vi "soundwave_generator_v06_complete_main.vi"() -> ()   [LabVIEW 2019]
uses:
  controls/Data.ctl
  <vilib>/sound2/lvsound2.llb/Sound Output Task ID.ctl
  controls/State.ctl
  <vilib>/sound2/lvsound2.llb/Sound Data Format.ctl
  <vilib>/sound2/lvsound2.llb/Sampling Mode.ctl
  <vilib>/Platform/TimedLoop/XDataNode/timing_clust.ctl
  <vilib>/Platform/TimedLoop/XDataNode/nitl_modes.ctl
  <vilib>/Platform/TimedLoop/XDataNode/wakeup.ctl
  add63f69-d936-4ba7-9212-3bb4b78ce241.vi
  global.vi
  <vilib>/sound2/lvsound2.llb/Sound File Read Open.vi
  <vilib>/sound2/lvsound2.llb/Sound File Read (DBL).vi
  <vilib>/Waveform/WDTOps.llb/WDT Waveform Duration DBL.vi
  <vilib>/sound2/lvsound2.llb/Sound Output Set Volume (Single).vi
  <vilib>/sound2/lvsound2.llb/Sound Output Write (DBL Single).vi
  <vilib>/platform/TimedLoop/XDataNode/XDataNode.xnode
  <vilib>/Platform/TimedLoop/XDataNode/XDNodeRunTimeDep.lvlib
panel:
  in  "Waiting time 2 [ms]":i32=1000
  in  "Waiting time 1 [ms]":i32=2000
  in  "# Repetitions":i32=3
  out "User Choice":string
  out "Real sound Duration [s] (Not Rounded)":dbl
  in  "Volume":dbl(slide)=50.0 min=0.0 max=100.0 step=1.0 scale=0.0..100.0
  out "Sound Duration [s]":dbl
  in  "Sound Samples Directory":path=path "D:/Scuola Superiore Sant'Anna/Neuro-Robotic Touch Laboratory - PhD Marian Statache - PhD Marian Statache/03 - HW & SW/Sound Psychophysical Protocol v3/sound_samples/2sec_352-00_396-00_412-50_440-00_469-33_495-00_528-00" caption="start path"
  out "Section 5":bool
  out "Section 4":bool
  out "Section 3":bool
  out "Section 1":bool
  in  "Saving Directory":path=path "D:/Scuola Superiore Sant'Anna/Neuro-Robotic Touch Laboratory - PhD Marian Statache - PhD Marian Statache/03 - HW & SW/Sound Psychophysical Protocol v3/trials"
  out "Sound 2":string
  out "Sound 1":string
  out "Remaining time":i32(slide) scale=-1.0..2000.0
  out "Remaining Time [ms]":i32
  out "Sound number":string
  in  "Start Button":bool
  out "Trial":i32=1 caption="Trial #:"
  in  "stop":bool
  # "1. Preliminary Settings"
  # "2. Start Protocol"
  # "3. Trial Info"
  # "4. User Choice"
  # "5. Protocol Termination"
  # "Dev. info"
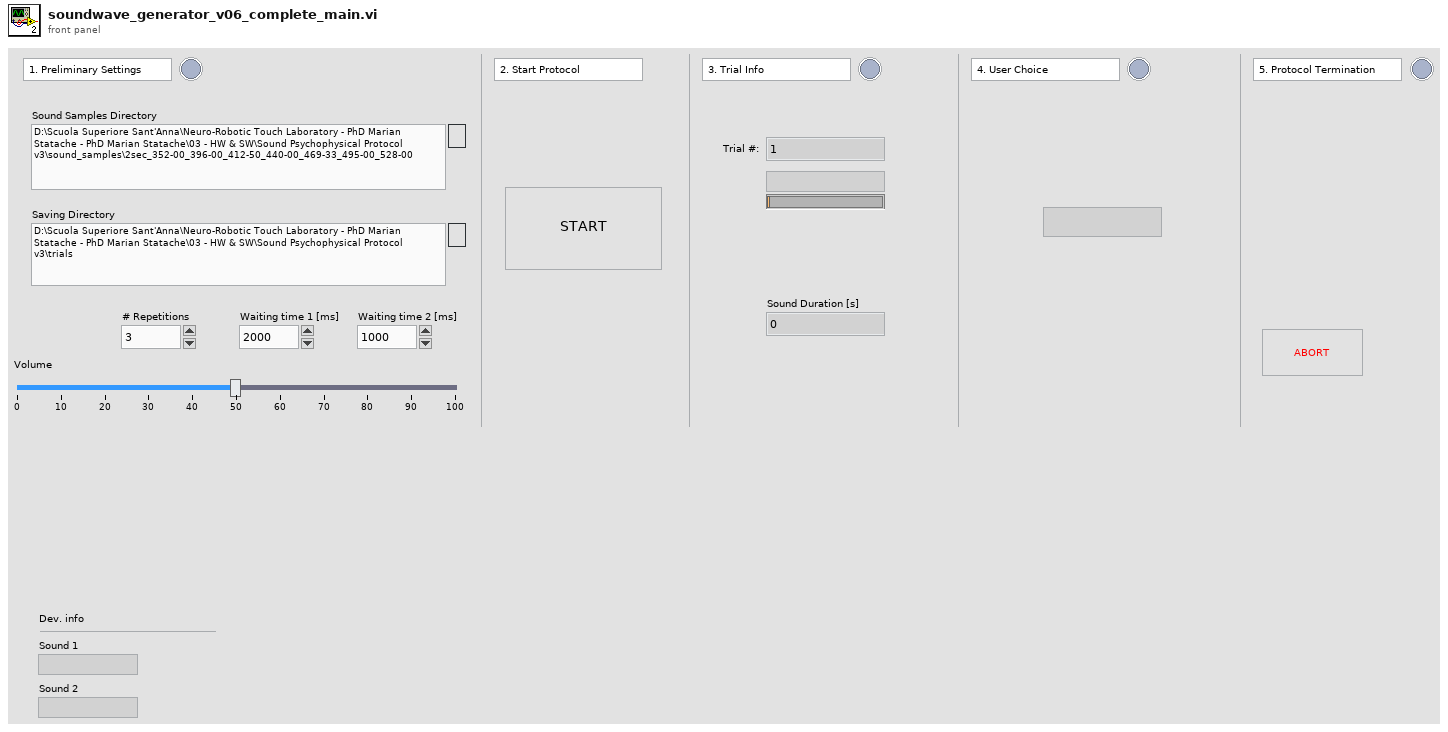
[diagram p1: front panel]
types:
  T1 = typedef "State.ctl" = enum16{"Initialize", "Wait for Start", "Preparation 1", "Preparation 2", "Start New Trial", "Wait S1", "Play Sound 1", "Wait S2", "Play Sound 2", "Wait for Answer", "Cleanup", "Exit"}
  T2 = typedef "Data.ctl" = cluster{"User VI Reference":refnum<vi>, "Output Text File Reference":refnum<file>, "#Sound Total Combinations ":i32, "Audio Task ID":T3, "Sound ID Combination Matrix":u8[][], "Sound Name Combination Matrix":string[][], "Sound Data Combination Matrix":waveform(dbl)[][], "Shuffled Array (Matrix Row Idxs)":i32[], "Sound 1 Data":waveform(dbl), "Sound 2 Data":waveform(dbl), "Repetitions idx":i32, "Combination idx":i32, "Repetition Flag":bool}
  T3 = typedef "Sound Output Task ID.ctl" = u32
  T4 = enum16{"open", "replace", "create", "open or create", "replace or create", "replace or create with confirmation"}
  T5 = typedef "Sound Data Format.ctl" = cluster{"sample rate (S/s)":dbl, "number of channels":i32, "bits per sample":i32}
  T6 = typedef "XDNodeRunTimeDep.lvlib/timing_clust.ctl" = cluster{"Expected End [f-1]":u64, "Actual End [f-1]":u64, "Finished Late? [f-1]":bool, "Expected End [i-1]":u64, "Actual End [i-1]":u64, "Finished Late? [i-1]":bool, "Expected Start [i]":u64, "Actual Start [i]":u64, "Expected Start [f]":u64, "Actual Start [f]":u64, "Source Name":string, "Structure Name":string, "Period":i64, "Deadline":i64, "Offset":i64, "Start":i64, "Priority":i32, "Timeout":i32, "Mode":T7, "Wakeup Reason":T8, "Error":errorcluster, "Source Type":string, "Secondary Source Type":string, "Global End Time":u64, "Global Start Time":u64, "Frame Duration":u64, "Iteration Duration":u64, "Assigned CPU":i32, "I/O Scan Engine Mode":u32}
  T7 = typedef "XDNodeRunTimeDep.lvlib/nitl_modes.ctl" = enum32{"No Change", "Process missed periods, maintain original phase", "Discard missed periods, maintain original phase", "Process missed periods, ignore original phase", "Discard missed periods, ignore original phase"}
  T8 = typedef "XDNodeRunTimeDep.lvlib/wakeup.ctl" = enum32{"Normal", "Aborted", "Asynchronous wakeup", "Timing source error", "Timed loop error", "Timeout"}
  T9 = typedef "Sampling Mode.ctl" = i32
  T10 = typedef "Sound File Refnum.ctl" = refnum<file>
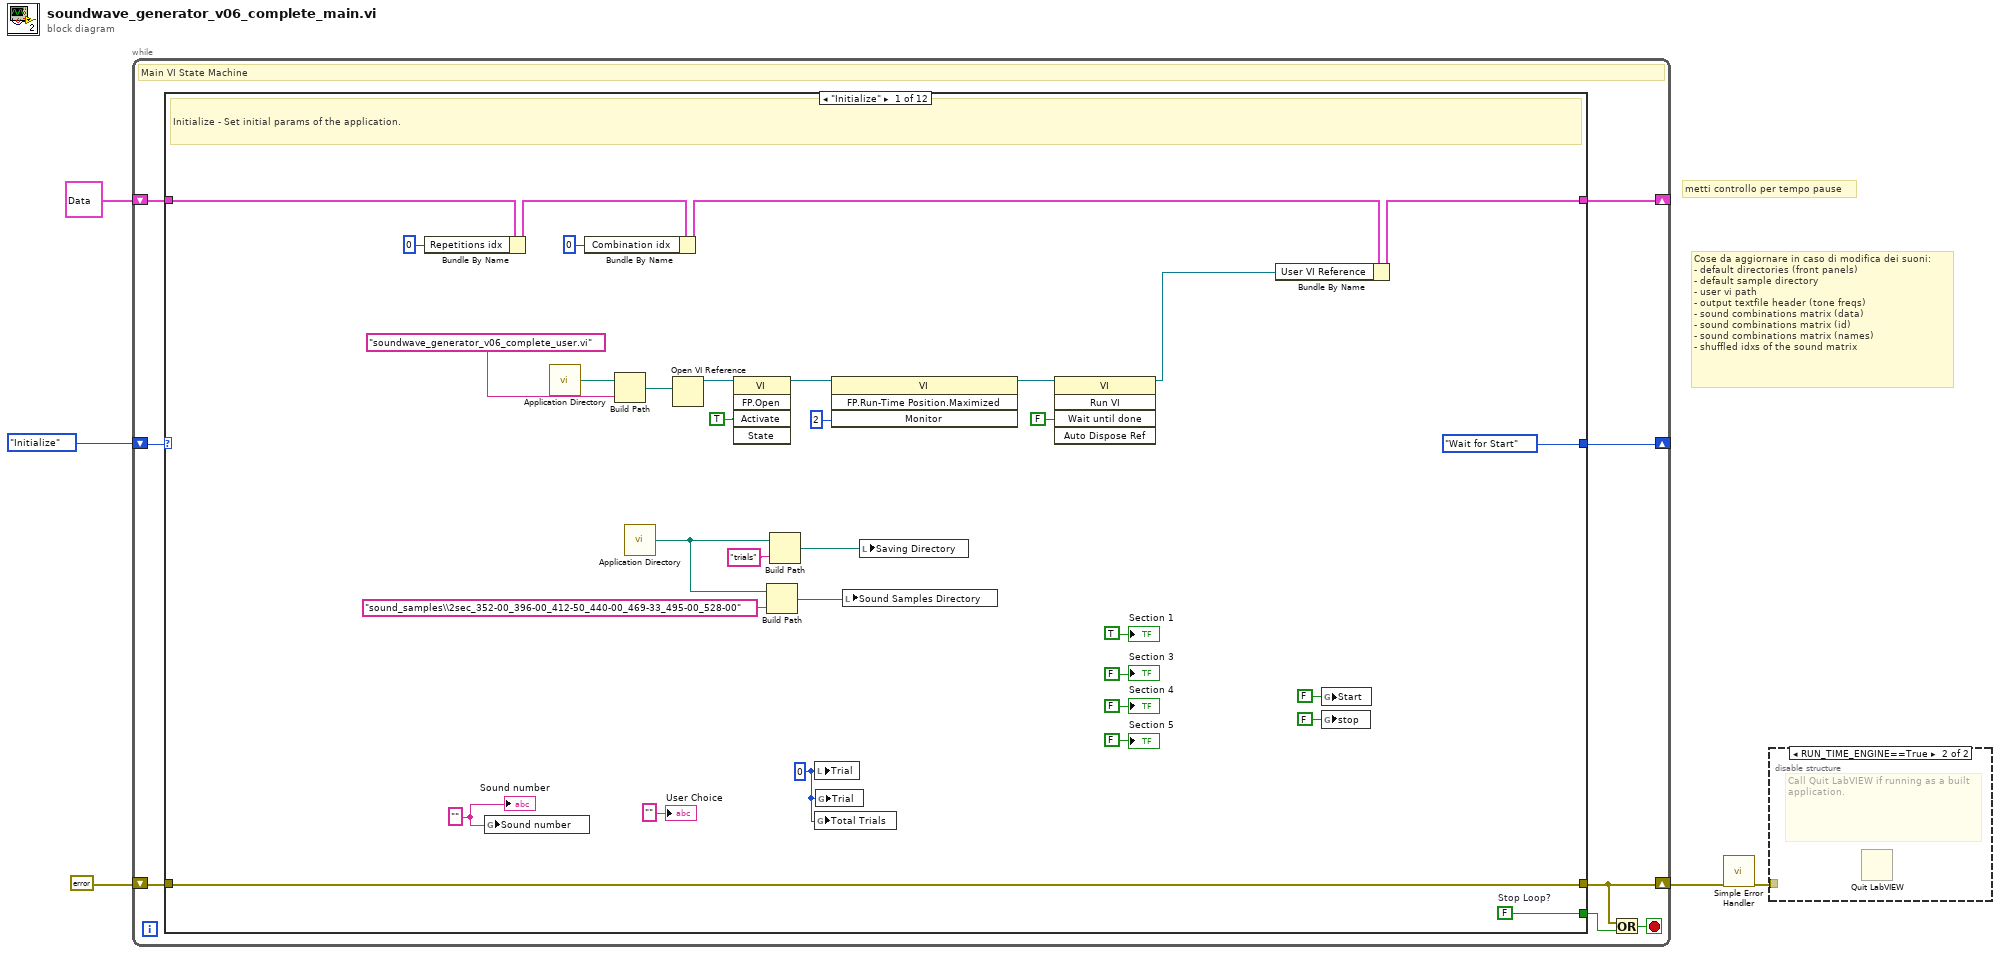
[diagram p0: block diagram]
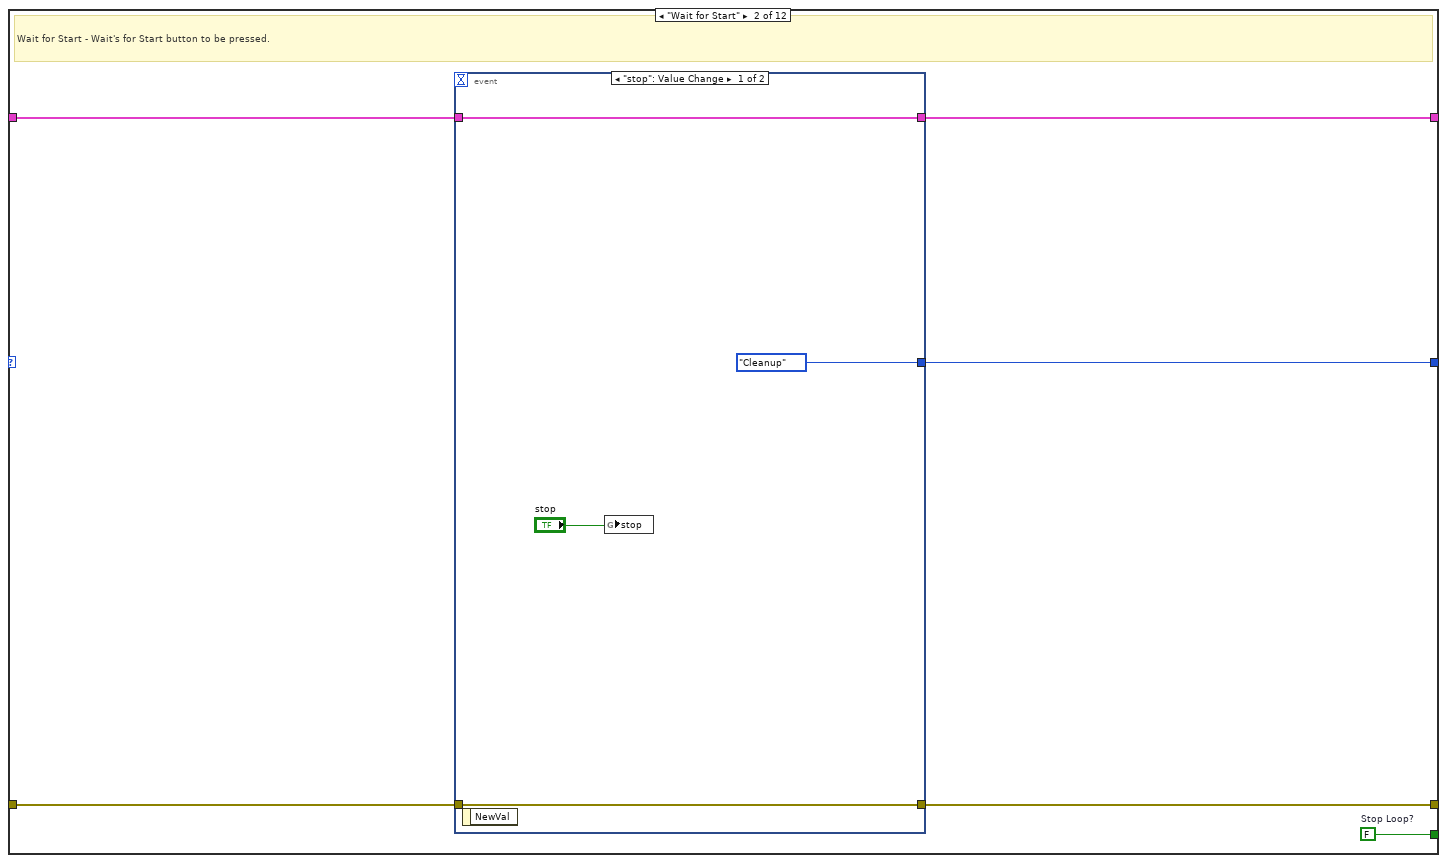
[diagram p3: hidden frame]
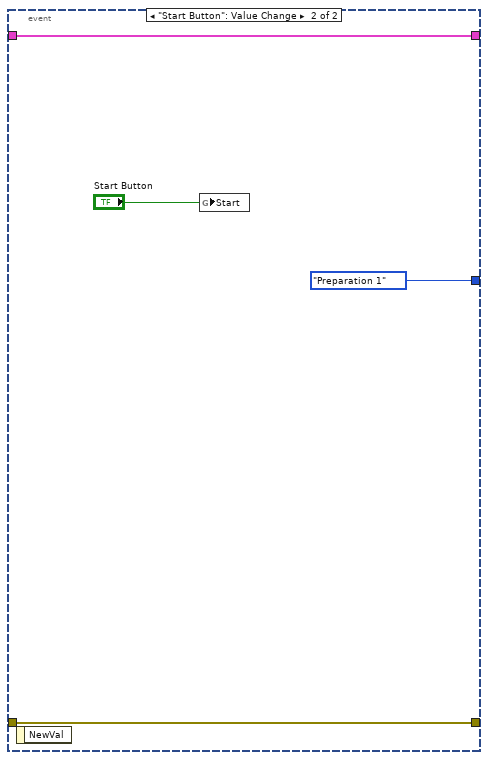
[diagram p4: hidden frame]
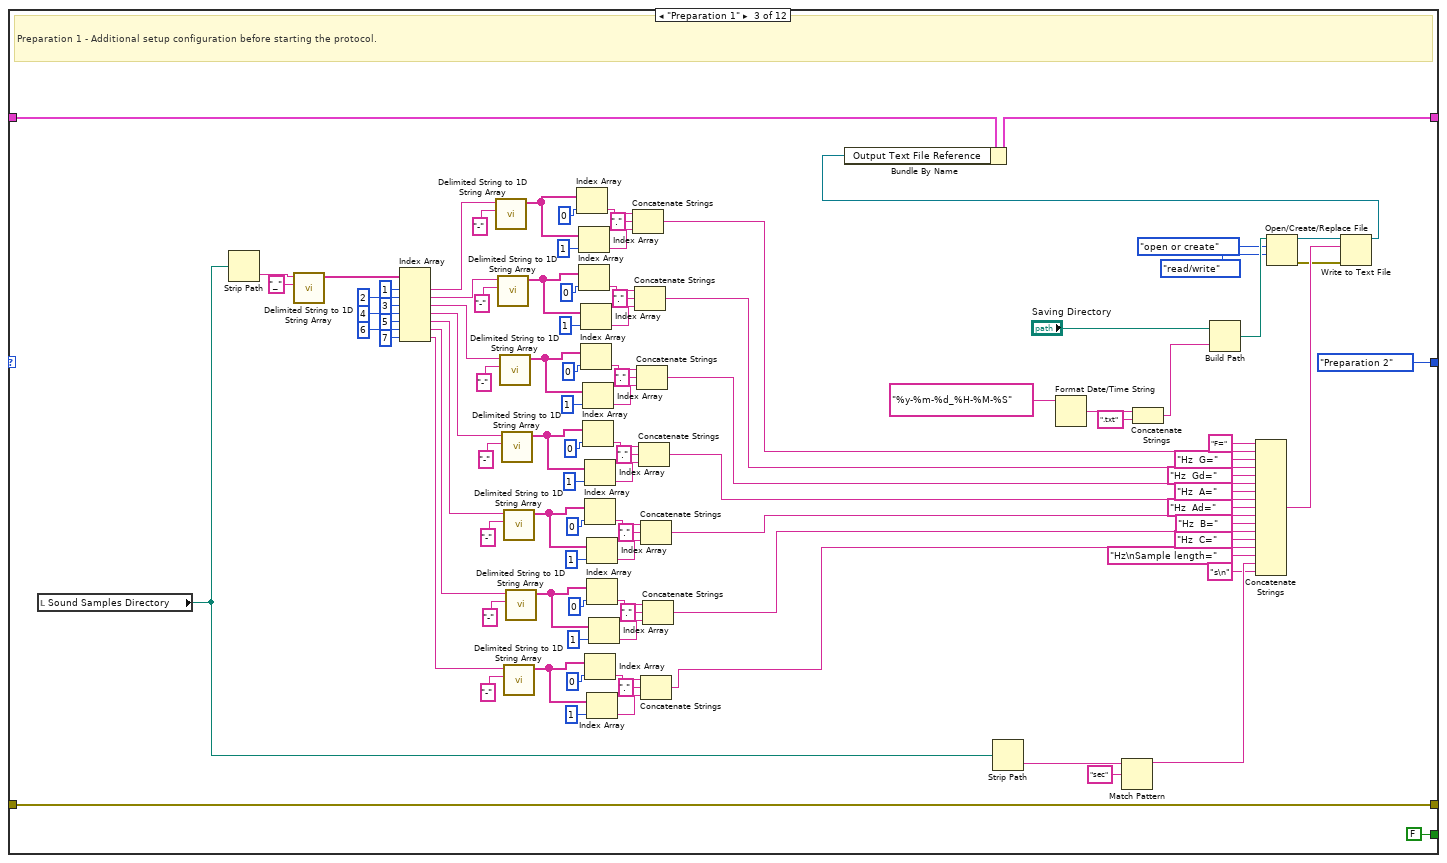
[diagram p5: hidden frame]
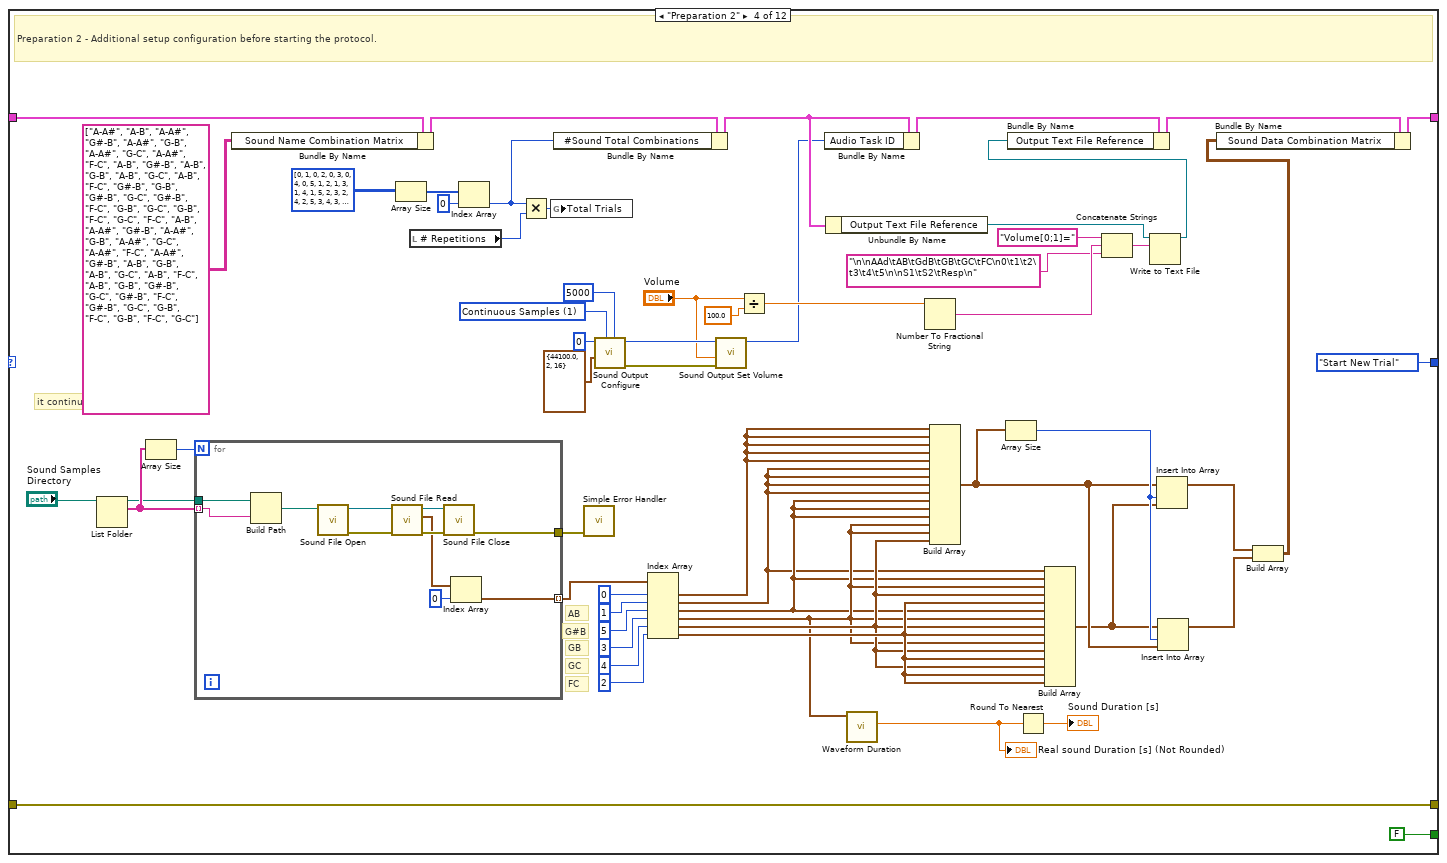
[diagram p6: hidden frame]
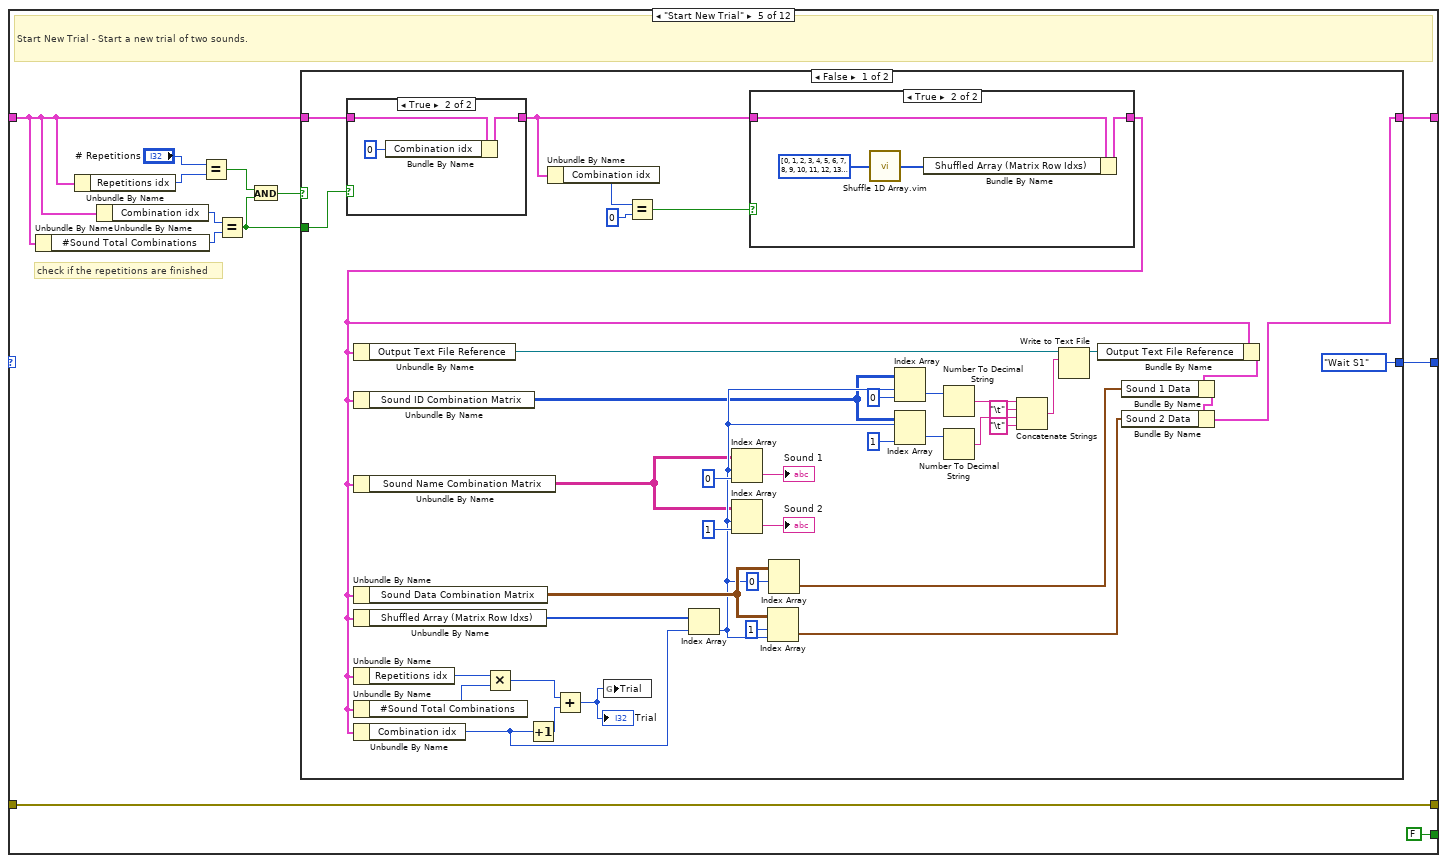
[diagram p7: hidden frame]
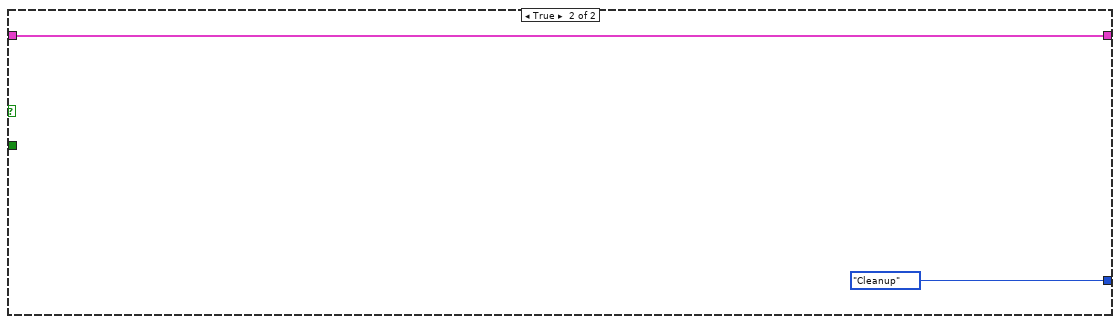
[diagram p10: hidden frame]
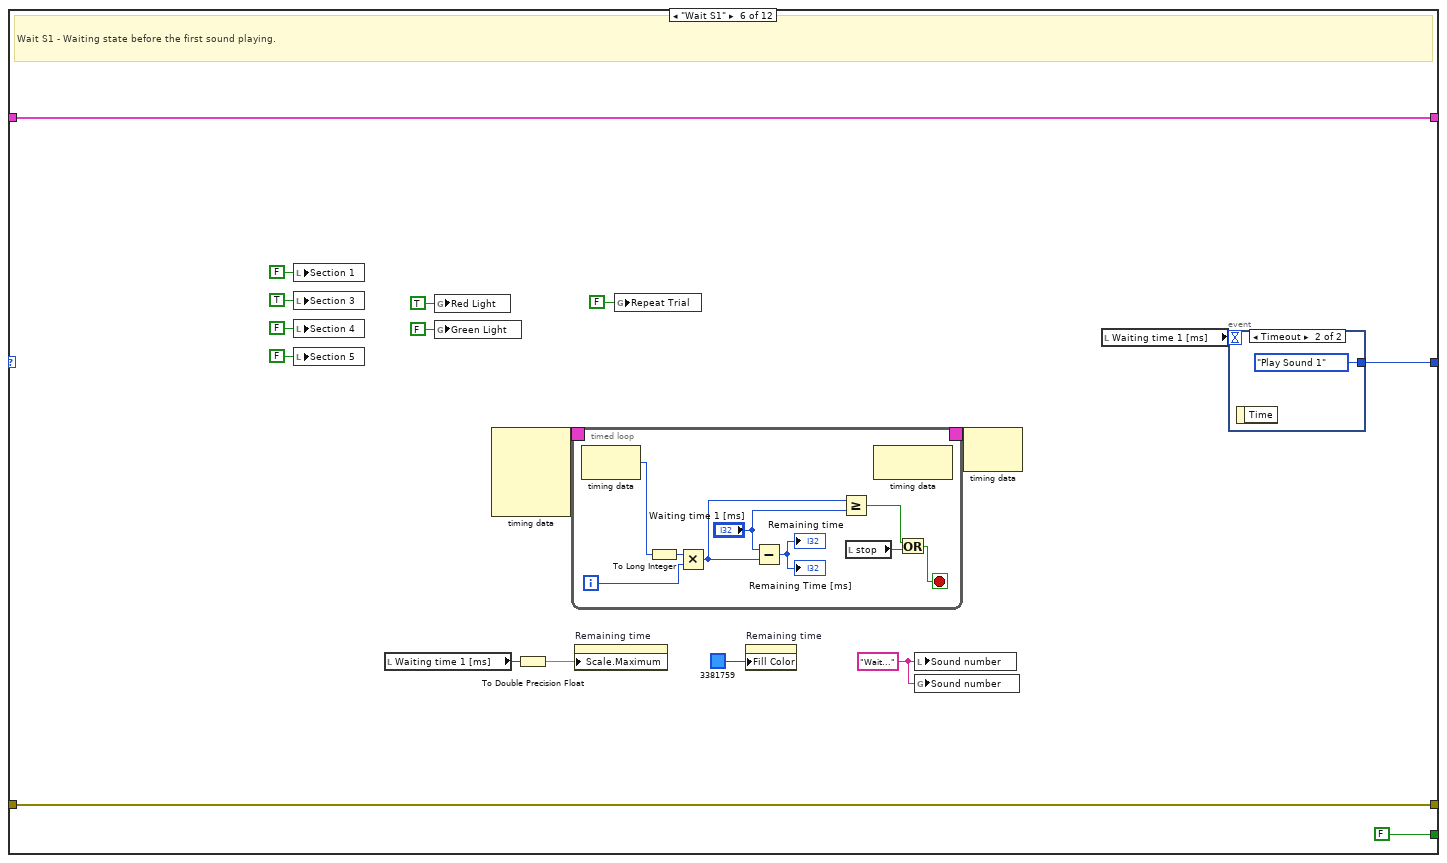
[diagram p11: hidden frame]
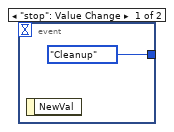
[diagram p12: hidden frame]
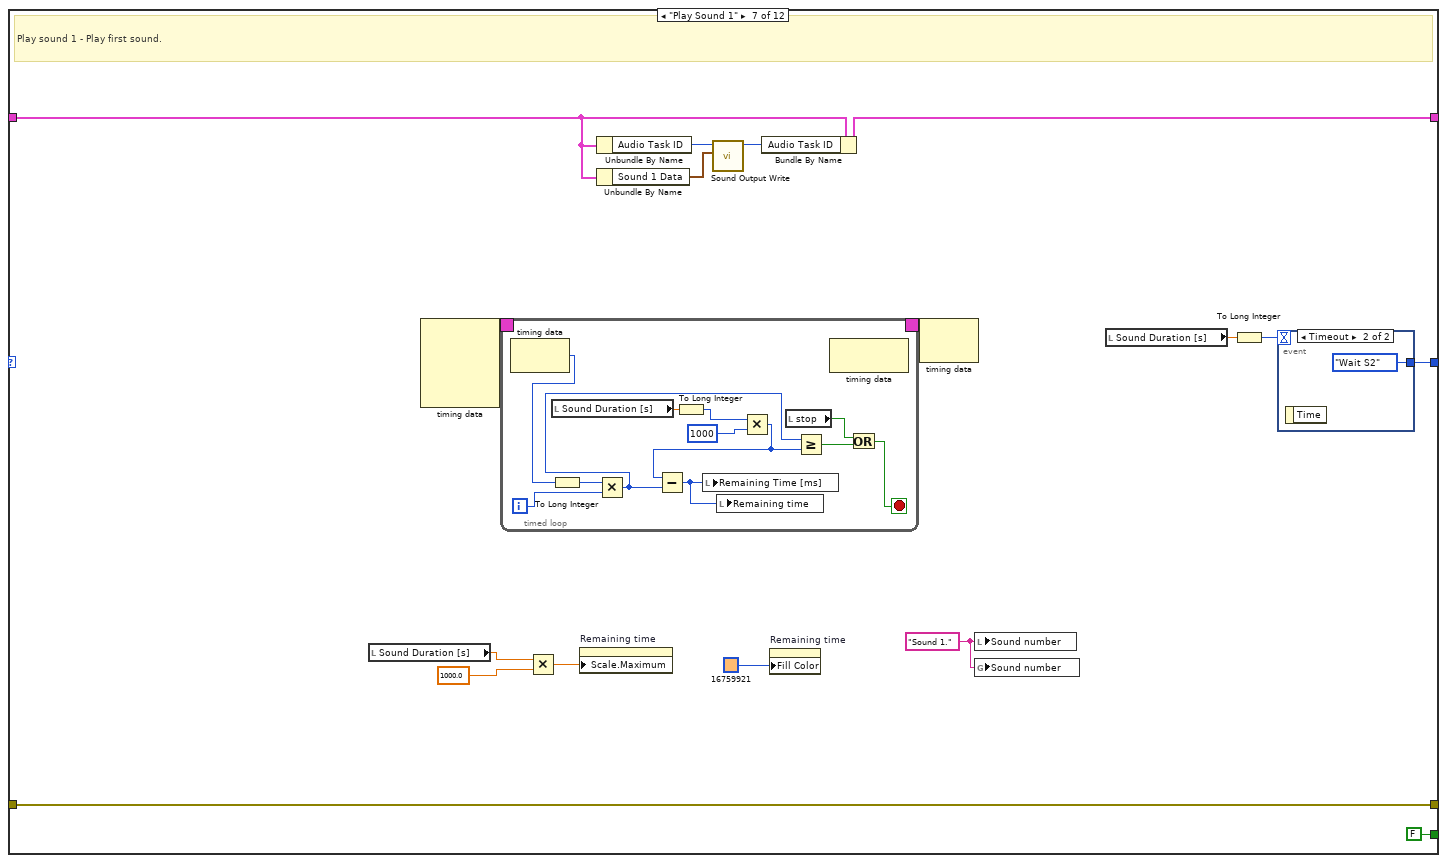
[diagram p13: hidden frame]
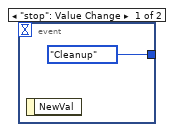
[diagram p14: hidden frame]
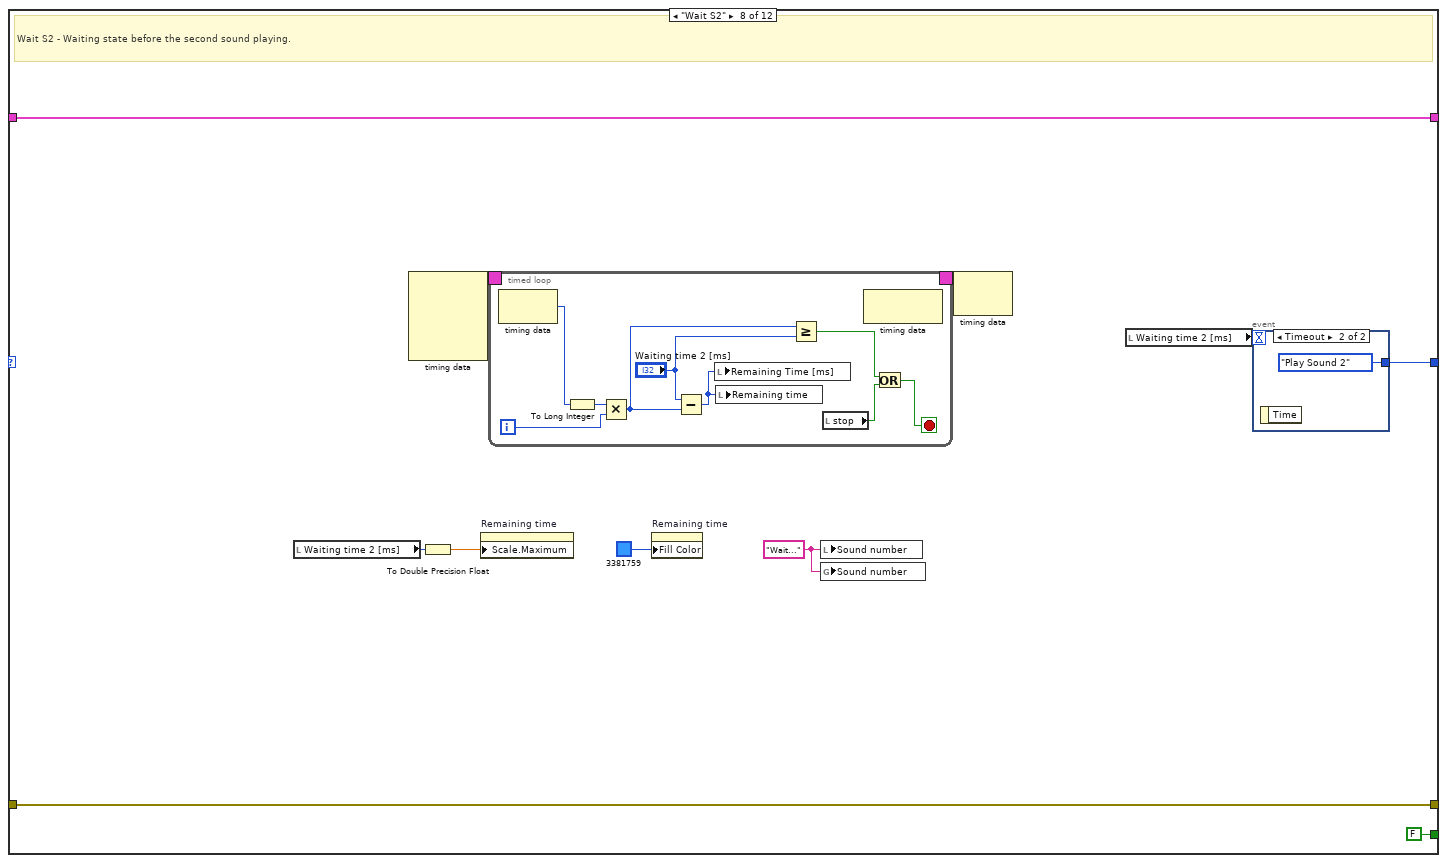
[diagram p15: hidden frame]
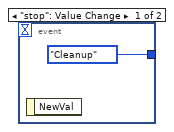
[diagram p16: hidden frame]
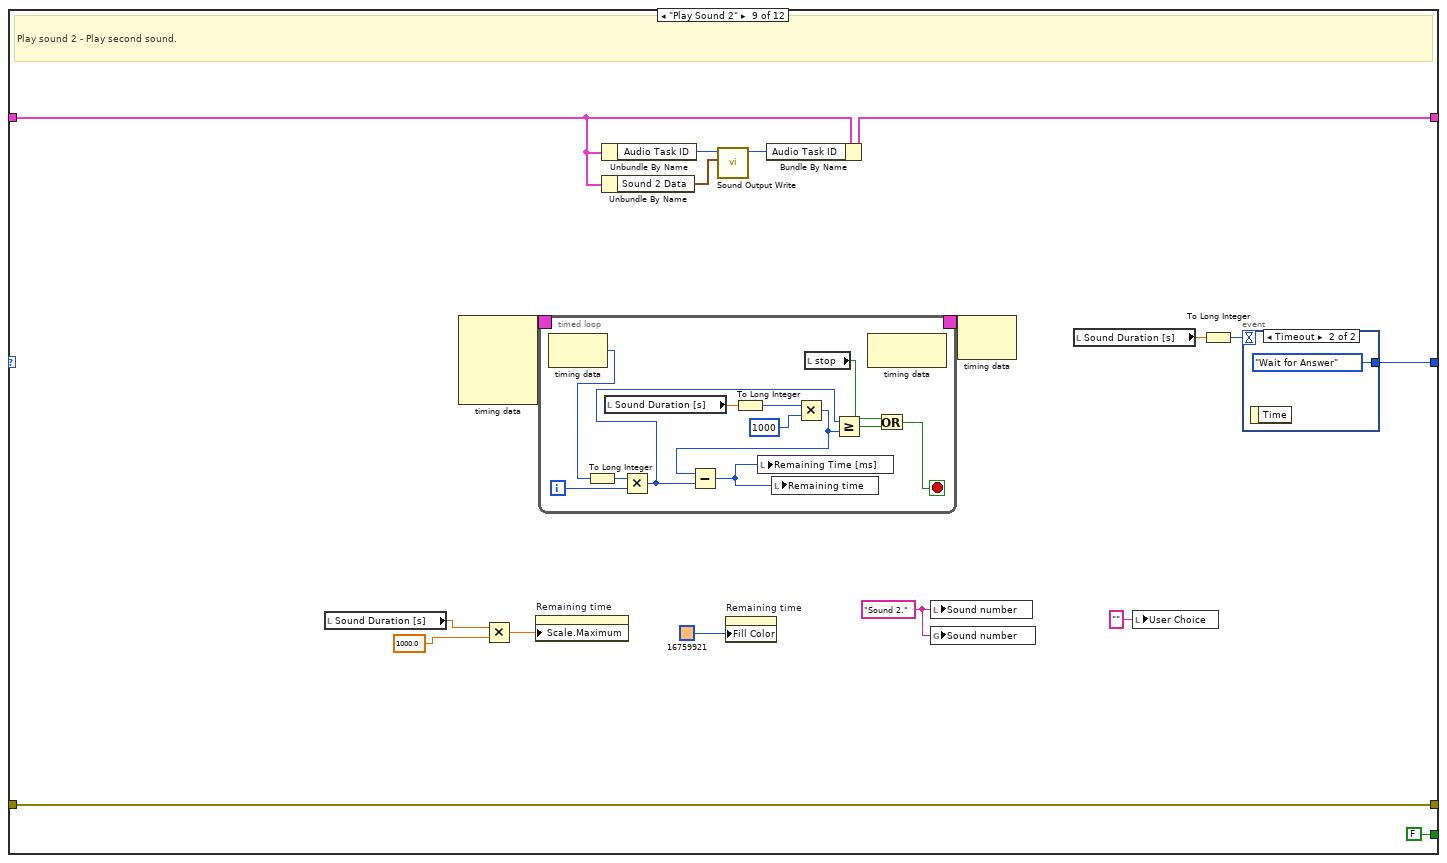
[diagram p17: hidden frame]
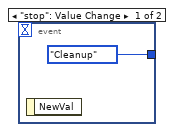
[diagram p18: hidden frame]
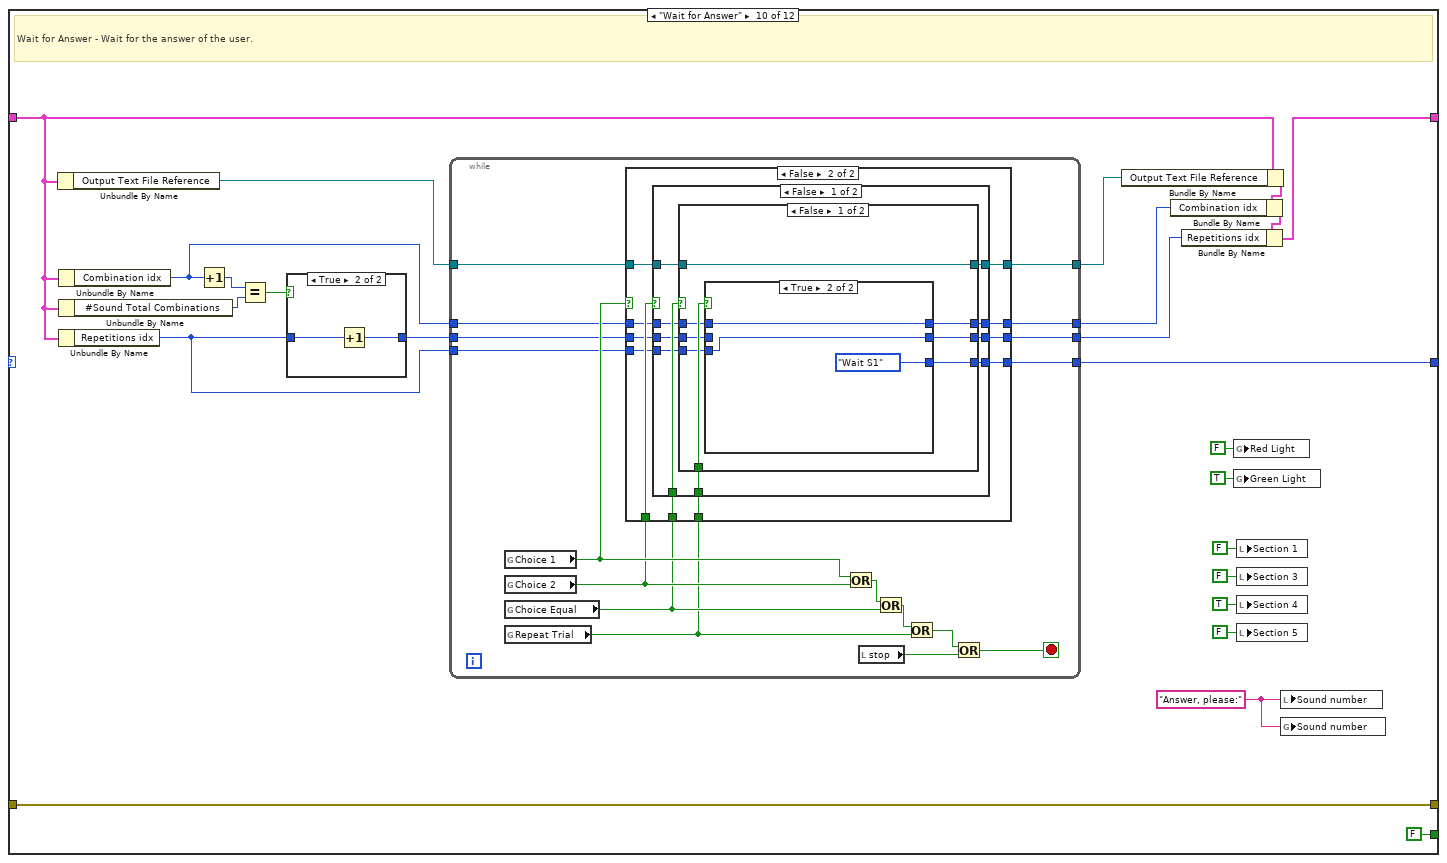
[diagram p19: hidden frame]
diagram:
  # "metti controllo per tempo pause"
  # "Cose da aggiornare in caso di modifica dei suoni:\n- default directories (front panels)\n- default sample directory\n- user vi path\n- output textfile header (tone freqs)\n- sound combinations matrix (data)\n- sound combinations matrix (id)\n- sound combinations matrix (names)\n- shuffled idxs of the sound matrix"
  n1 = while {
    shift-right: [w12] -> _
    shift-left: State."Initialize" ("States") -> [w13]
    shift-right: [w10] -> _
    shift-left: T2 {"User VI Reference"=refnum, "Output Text File Reference"=refnum, "#Sound Total Combinations "=0, "Audio Task ID"=0, "Sound ID Combination Matrix"=[[0, 1], [0, 2], [0, 3], [0, 4], [0, 5], [1, 2], [1, 3], [1, 4], [1, 5], [2, 3], [2, 4], [2, 5], [3, 4], [3, 5], [4, 5], [1, 0], [2, 0], [3, 0], [4, 0], [5, 0], [2, 1], [3, 1], [4, 1], [5, 1], [3, 2], [4, 2], [5, 2], [4, 3], [5, 3], [5, 4]], "Sound Name Combination Matrix"=[["A-A#", "A-B"], ["A-A#", "G#-B"], ["A-A#", "G-B"], ["A-A#", "G-C"], ["A-A#", "F-C"], ["A-B", "G#-B"], ["A-B", "G-B"], ["A-B", "G-C"], ["A-B", "F-C"], ["G#-B", "G-B"], ["G#-B", "G-C"], ["G#-B", "F-C"], ["G-B", "G-C"], ["G-B", "F-C"], ["G-C", "F-C"], ["A-B", "A-A#"], ["G#-B", "A-A#"], ["G-B", "A-A#"], ["G-C", "A-A#"], ["F-C", "A-A#"], ["G#-B", "A-B"], ["G-B", "A-B"], ["G-C", "A-B"], ["F-C", "A-B"], ["G-B", "G#-B"], ["G-C", "G#-B"], ["F-C", "G#-B"], ["G-C", "G-B"], ["F-C", "G-B"], ["F-C", "G-C"]], "Sound Data Combination Matrix"=[], "Shuffled Array (Matrix Row Idxs)"=[], "Sound 1 Data"={"t0"=timestamp(0 s since 1904-01-01), "dt"=1.0, "Y"=[]}, "Sound 2 Data"={"t0"=timestamp(0 s since 1904-01-01), "dt"=1.0, "Y"=[]}, "Repetitions idx"=0, "Combination idx"=0, "Repetition Flag"=FALSE} ("Data") -> [w11]
    shift-right: [w6] -> w4
    shift-left: errorcluster {"status"=FALSE, "code"=0, "source"=""} ("error constant") -> [w9]
    stop <- w7 stop-if-true
    # "Main VI State Machine"
    n2 = case shown="\"Initialize\"" w13 {
      tunnel: [State."Wait for Start" ("States") w52 State."Preparation 2" ("(Value Not Used)") State."Start New Trial" ("States") w234 w305 w345 w370 w396 w443 State."Exit" ("States") w554] -> w12
      tunnel: [w46 w51 FALSE ("Stop Loop?") FALSE ("Stop Loop?") FALSE ("Stop Loop?") FALSE ("Stop Loop?") FALSE ("Stop Loop?") FALSE ("Stop Loop?") FALSE ("Stop Loop?") FALSE ("Stop Loop?") FALSE ("Stop Loop?") w553] -> w8
      tunnel: w11 -> [w20 w50 w63 w176 w235 w306 w335 w377 w398 w436 w536 w551]
      tunnel: [w45 w49 w62 w218 w236 w306 w334 w377 w397 w437 w536 w551] -> w10
      tunnel: w9 -> [w44 w48 w163 w220 w244 w313 w347 w376 w411 w454 w549 w552]
      tunnel: [w44 w47 w163 w220 w244 w313 w347 w376 w411 w454 w549 w552] -> w6
      frame "Initialize" {
        w28 = 0 ("Trial")
        w40 = "" ("String")
        w46 = FALSE  # Stop Loop?
        # "Initialize - Set initial params of the application."
        n3 = Bundle By Name(cluster=w20, "Repetitions idx"=0) -> (w19:T2)
        n4 = global write "global.vi" "Sound number"(w40) -> ()
        n5 = call <vilib>:"Application Directory.vi"() -> ("Application Directory"=w35:path)
        n6 = Bundle By Name(cluster=w19, "Combination idx"=0) -> (w18:T2)
        n7 = Build Path(base path=w35, name or relative path="soundwave_generator_v06_complete_user.vi") -> (appended path=w34:path)
        n8 = call <vilib>:"Application Directory.vi"() -> ("Application Directory"=w43:path)
        n9 = Open VI Reference(vi path=w34) -> (vi reference=w33:refnum<vi>)  [unwired: 5 in, 1 out]
        n10 = invoke class="VI" method="FP.Open"(reference=w33, "Activate"=TRUE ("Activate?")) -> (reference out=w36:refnum<vi>)  [unwired: 3 in, 4 out]
        n11 = Build Path(base path=w43, name or relative path="sound_samples\\2sec_352-00_396-00_412-50_440-00_469-33_495-00_528-00") -> (appended path=w42:path)
        n12 = Build Path(base path=w43, name or relative path="trials") -> (appended path=w41:path)
        n13 = local write "Trial"(w28) -> ()
        n14 = global write "global.vi" "Total Trials"(w28) -> ()
        n15 = global write "global.vi" "Trial"(w28) -> ()
        n16 = invoke class="VI" method="FP.Run-Time Position.Maximized"(reference=w36, "Monitor"=i16 2) -> (reference out=w37:refnum<vi>)  [unwired: 2 in, 3 out]
        n17 = local write "Sound Samples Directory"(w42) -> ()
        n18 = local write "Saving Directory"(w41) -> ()
        n19 = invoke class="VI" method="Run VI"(reference=w37, "Wait until done"=FALSE ("Wait Until Done")) -> (reference out=w22:refnum<vi>)  [unwired: 3 in, 4 out]
        n20 = Bundle By Name(cluster=w18, "User VI Reference"=w22) -> (w45:T2)
        n21 = global write "global.vi" "Start"(FALSE ("Start")) -> ()
        n22 = global write "global.vi" "stop"(FALSE ("stop")) -> ()
        "Sound number" <- w40
        "Section 1" <- TRUE ("Section 1")
        "Section 3" <- FALSE ("Section 3")
        "Section 4" <- FALSE ("Section 4")
        "Section 5" <- FALSE ("Section 5")
        "User Choice" <- "" ("User Choice")
      }
      frame "Wait for Start" {
        w51 = FALSE  # Stop Loop?
        # "Wait for Start - Wait's for Start button to be pressed."
        n23 = event shown="[0] \"stop\": Value Change" {
          selector: _ -> [_ _]
          dyn-events: _ -> [_ _]
          timeout: _ -> [_ _]
          tunnel: [State."Cleanup" ("States") State."Preparation 1" ("States")] -> w52
          tunnel: w50 -> [w56 w60]
          tunnel: [w56 w60] -> w49
          tunnel: w48 -> [w55 w59]
          tunnel: [w55 w59] -> w47
          event "stop": Value Change {
            n24 = event-data() -> ()  [unwired: 1 in, 1 out]
            n25 = global write "global.vi" "stop"("stop") -> ()
          }
          event "Start Button": Value Change {
            n26 = event-data() -> ()  [unwired: 1 in, 1 out]
            n27 = global write "global.vi" "Start"("Start Button") -> ()
          }
        }
      }
      frame "Preparation 1" {
        # "Preparation 1 - Additional setup configuration before starting the protocol."
        n28 = local read "Sound Samples Directory"() -> (w61:path)
        n29 = Strip Path(path=w61) -> (name=w129:string)  [unwired: 1 out]
        n30 = call <vilib>:"Delimited String to 1D String Array.vi"("delimiter"="_", "delimited string"=w129) -> ("string array"=w130:string[])  [unwired: 9 in]
        n31 = Index Array(array=w130, index #1=1 ("index"), index #2=2 ("index"), index #3=3 ("index"), index #4=4 ("index"), index #5=5 ("index"), index #6=6 ("index"), index #7=7 ("index")) -> (element #1=w131:string, element #2=w146:string, element #3=w147:string, element #4=w148:string, element #5=w149:string, element #6=w154:string, element #7=w158:string)
        n32 = call <vilib>:"Delimited String to 1D String Array.vi"("delimiter"="-", "delimited string"=w131) -> ("string array"=w132:string[])  [unwired: 9 in]
        n33 = call <vilib>:"Delimited String to 1D String Array.vi"("delimiter"="-", "delimited string"=w146) -> ("string array"=w135:string[])  [unwired: 9 in]
        n34 = call <vilib>:"Delimited String to 1D String Array.vi"("delimiter"="-", "delimited string"=w147) -> ("string array"=w138:string[])  [unwired: 9 in]
        n35 = call <vilib>:"Delimited String to 1D String Array.vi"("delimiter"="-", "delimited string"=w148) -> ("string array"=w141:string[])  [unwired: 9 in]
        n36 = call <vilib>:"Delimited String to 1D String Array.vi"("delimiter"="-", "delimited string"=w149) -> ("string array"=w144:string[])  [unwired: 9 in]
        n37 = call <vilib>:"Delimited String to 1D String Array.vi"("delimiter"="-", "delimited string"=w158) -> ("string array"=w156:string[])  [unwired: 9 in]
        n38 = call <vilib>:"Delimited String to 1D String Array.vi"("delimiter"="-", "delimited string"=w154) -> ("string array"=w151:string[])  [unwired: 9 in]
        n39 = Index Array(array=w132, index=0) -> (element=w128:string)
        n40 = Index Array(array=w132, index=1) -> (element=w133:string)
        n41 = Index Array(array=w135, index=0) -> (element=w136:string)
        n42 = Index Array(array=w135, index=1) -> (element=w134:string)
        n43 = Index Array(array=w138, index=0) -> (element=w139:string)
        n44 = Index Array(array=w138, index=1) -> (element=w137:string)
        n45 = Index Array(array=w141, index=0) -> (element=w142:string)
        n46 = Index Array(array=w141, index=1) -> (element=w140:string)
        n47 = Index Array(array=w144, index=0) -> (element=w145:string)
        n48 = Index Array(array=w156, index=0) -> (element=w157:string)
        n49 = Index Array(array=w144, index=1) -> (element=w143:string)
        n50 = Index Array(array=w151, index=0) -> (element=w152:string)
        n51 = Index Array(array=w156, index=1) -> (element=w155:string)
        n52 = Index Array(array=w151, index=1) -> (element=w150:string)
        n53 = Concatenate Strings(w128, "." ("string"), w133) -> (w121:string)
        n54 = Concatenate Strings(w136, "." ("string"), w134) -> (w122:string)
        n55 = Concatenate Strings(w139, "." ("string"), w137) -> (w123:string)
        n56 = Concatenate Strings(w142, "." ("string"), w140) -> (w124:string)
        n57 = Concatenate Strings(w145, "." ("string"), w143) -> (w125:string)
        n58 = Concatenate Strings(w157, "." ("string"), w155) -> (w160:string)
        n59 = Concatenate Strings(w152, "." ("string"), w150) -> (w153:string)
        n60 = Strip Path(path=w61) -> (name=w126:string)  [unwired: 1 out]
        n61 = Format Date/Time String(time format string (%c)="%y-%m-%d_%H-%M-%S") -> (date/time string=w115:string)  [unwired: 2 in]
        n62 = Match Pattern(string=w126, regular expression="sec") -> (before substring=w159:string)  [unwired: 1 in, 3 out]
        n63 = Concatenate Strings(w115, ".txt" ("string")) -> (w119:string)
        n64 = Build Path(base path="Saving Directory", name or relative path=w119) -> (appended path=w120:path)
        n65 = Concatenate Strings("F=" ("string"), w121, "Hz  G=" ("string"), w122, "Hz  Gd=" ("string"), w123, "Hz  A=" ("string"), w124, "Hz  Ad=" ("string"), w125, "Hz  B=" ("string"), w153, "Hz  C=" ("string"), w160, "Hz\nSample length=" ("string"), w159, "s\n" ("string")) -> (w127:string)
        n66 = Open/Create/Replace File(file path (use dialog)=w120, operation (0:open)=T4."open or create", access (0:read/write)=enum16{"read/write", "read-only", "write-only"}."read/write") -> (refnum out=w116:refnum<file>, error out=w117:errorcluster)  [unwired: 3 in, 1 out]
        n67 = Write to Text File(file (use dialog)=w116, text=w127, error in=w117) -> (refnum out=w64:refnum<file>)  [unwired: 1 in, 2 out]
        n68 = Bundle By Name(cluster=w63, "Output Text File Reference"=w64) -> (w62:T2)
      }
      frame "Preparation 2" {
        w169 = T9 1 items=["Finite Samples", "Continuous Samples"] ("sample mode")
        # "it continues..."
        # "G#B"
        # "AB"
        # "GB"
        # "GC"
        # "FC"
        # "Preparation 2 - Additional setup configuration before starting the protocol."
        n69 = List Folder(path="Sound Samples Directory") -> (path out=w201:path, filenames=w202:string[])  [unwired: 3 in, 2 out]
        n70 = Array Size(array=w202) -> (size(s)=w203:i32)
        n71 = for {
          N: w203 -> [_]
          tunnel: w201 -> [w231]
          tunnel: w202 -> [w232] mode=indexing
          tunnel: [w225] -> w204
          tunnel: [w222] -> w205 mode=indexing
          n72 = Build Path(base path=w231, name or relative path=w232) -> (appended path=w226:path)
          n73 = call-poly <vilib>:"Sound File Open.vi"("path"=w226) -> ("error out"=w230:errorcluster, "sound file refnum"=w229:T10)  [unwired: 9 in]
          n74 = call-poly <vilib>:"Sound File Read.vi"("error in (no error)"=w230, "sound file refnum"=w229) -> ("error out"=w228:errorcluster, "data"=w223:waveform(dbl)[], "sound file refnum out"=w227:T10)  [unwired: 5 in, 2 out]
          n75 = call <vilib>:"Sound File Close.vi"("error in (no error)"=w228, "sound file refnum"=w227) -> ("error out"=w225:errorcluster)  [unwired: 9 in]
          n76 = Index Array(array=w223, index=0) -> (element=w222:waveform(dbl))
        }
        n77 = Bundle By Name(cluster=w176, "Sound Name Combination Matrix"=string[][] [["A-A#", "A-B"], ["A-A#", "G#-B"], ["A-A#", "G-B"], ["A-A#", "G-C"], ["A-A#", "F-C"], ["A-B", "G#-B"], ["A-B", "G-B"], ["A-B", "G-C"], ["A-B", "F-C"], ["G#-B", "G-B"], ["G#-B", "G-C"], ["G#-B", "F-C"], ["G-B", "G-C"], ["G-B", "F-C"], ["G-C", "F-C"], ["A-B", "A-A#"], ["G#-B", "A-A#"], ["G-B", "A-A#"], ["G-C", "A-A#"], ["F-C", "A-A#"], ["G#-B", "A-B"], ["G-B", "A-B"], ["G-C", "A-B"], ["F-C", "A-B"], ["G-B", "G#-B"], ["G-C", "G#-B"], ["F-C", "G#-B"], ["G-C", "G-B"], ["F-C", "G-B"], ["F-C", "G-C"]] ("Sound name")) -> (w173:T2)
        n78 = Array Size(array=u8[][] [[0, 1], [0, 2], [0, 3], [0, 4], [0, 5], [1, 2], [1, 3], [1, 4], [1, 5], [2, 3], [2, 4], [2, 5], [3, 4], [3, 5], [4, 5], [1, 0], [2, 0], [3, 0], [4, 0], [5, 0], [2, 1], [3, 1], [4, 1], [5, 1], [3, 2], [4, 2], [5, 2], [4, 3], [5, 3], [5, 4]] ("Array")) -> (size(s)=w180:i32[])
        n79 = local read "# Repetitions"() -> (w174:i32)
        n80 = Index Array(array=w180, index=0) -> (element=w172:i32)
        n81 = Multiply(x=w172, y=w174) -> (x*y=w179:i32)
        n82 = global write "global.vi" "Total Trials"(w179) -> ()
        n83 = Bundle By Name(cluster=w173, "#Sound Total Combinations"=w172) -> (w166:T2)
        n84 = call <vilib>:"Simple Error Handler.vi"("error in (no error)"=w204) -> ()  [unwired: 4 in, 5 out]
        n85 = call <vilib>:"Sound Output Configure.vi"("number of samples/ch"=5000, "sample mode"=w169, "sound format"=T5 {"sample rate (S/s)"=44100.0, "number of channels"=2, "bits per sample"=16}, "device ID"=u32 0) -> ("error out"=w190:errorcluster, "task ID"=w191:T3)  [unwired: 6 in]
        n86 = Index Array(array=w205, index #1=0 ("index"), index #2=1 ("index"), index #3=5 ("index"), index #4=3 ("index"), index #5=4 ("index"), index #6=2 ("index")) -> (element #1=w192:waveform(dbl), element #2=w211:waveform(dbl), element #3=w212:waveform(dbl), element #4=w213:waveform(dbl), element #5=w214:waveform(dbl), element #6=w215:waveform(dbl))
        n87 = call-poly <vilib>:"Sound Output Set Volume.vi"("error in (no error)"=w190, "volume"="Volume", "task ID"=w191) -> ("task ID out"=w165:T3)  [unwired: 7 in, 1 out]
        n88 = Divide(x="Volume", y=100.0) -> (x/y=w186:dbl)
        n89 = Bundle By Name(cluster=w166, "Audio Task ID"=w165) -> (w164:T2)
        n90 = Unbundle By Name(w166) -> ("Output Text File Reference"=w183:refnum<file>)
        n91 = call-poly <vilib>:"Waveform Duration.vi"("waveform in"=w213) -> ("duration"=w207:dbl)  [unwired: 8 in, 2 out]
        "Real sound Duration [s] (Not Rounded)" <- w207
        n92 = Number To Fractional String(number=w186) -> (F-format string=w189:string)  [unwired: 3 in]
        n93 = Build Array(w192, w192, w192, w192, w192, w211, w211, w211, w211, w212, w212, w212, w213, w213, w214) -> (w216:waveform(dbl)[])
        n94 = Array Size(array=w216) -> (size(s)=w217:i32)
        n95 = Round To Nearest(number=w207) -> (nearest integer value=→"Sound Duration [s]":dbl)
        n96 = Build Array(w211, w212, w213, w214, w215, w212, w213, w214, w215, w213, w214, w215, w214, w215, w215) -> (w208:waveform(dbl)[])
        n97 = Concatenate Strings("Volume[0;1]=" ("string"), w189, "\n\nAAd\tAB\tGdB\tGB\tGC\tFC\n0\t1\t2\t3\t4\t5\n\nS1\tS2\tResp\n" ("text")) -> (w188:string)
        n98 = Write to Text File(file (use dialog)=w183, text=w188) -> (refnum out=w182:refnum<file>)  [unwired: 2 in, 2 out]
        n99 = Bundle By Name(cluster=w164, "Output Text File Reference"=w182) -> (w181:T2)
        n100 = Insert Into Array(array=w216, index=w217, new element=w208) -> (w209:waveform(dbl)[])
        n101 = Insert Into Array(array=w208, index=w217, new element=w216) -> (w210:waveform(dbl)[])
        n102 = Build Array(w209, w210) -> (w194:waveform(dbl)[][])
        n103 = Bundle By Name(cluster=w181, "Sound Data Combination Matrix"=w194) -> (w218:T2)
      }
      frame "Start New Trial" {
        # "check if the repetitions are finished"
        # "Start New Trial - Start a new trial of two sounds."
        n104 = Unbundle By Name(w235) -> ("#Sound Total Combinations"=w241:i32)
        n105 = Unbundle By Name(w235) -> ("Repetitions idx"=w242:i32)
        n106 = Unbundle By Name(w235) -> ("Combination idx"=w238:i32)
        n107 = Equal?(x="# Repetitions", y=w242) -> (x = y?=w240:bool)
        n108 = Equal?(x=w238, y=w241) -> (x = y?=w237:bool)
        n109 = And(x=w240, y=w237) -> (x .and. y?=w239:bool)
        n110 = case shown="False" w239 {
          tunnel: [w279 w296] -> w236
          tunnel: w235 -> [w283 w296]
          tunnel: [State."Wait S1" ("States") State."Cleanup" ("States")] -> w234
          tunnel: w237 -> [w284 _]
          frame False {
            n111 = case shown="True" w284 {
              tunnel: [w286 w288] -> w282
              tunnel: w283 -> [w286 w289]
              frame False {
              }
              frame True {
                n112 = Bundle By Name(cluster=w289, "Combination idx"=0) -> (w288:T2)
              }
            }
            n113 = Unbundle By Name(w282) -> ("Combination idx"=w281:i32)
            n114 = Equal?(x=w281, y=0) -> (x = y?=w277:bool)
            n115 = case shown="True" w277 {
              tunnel: [w290 w292] -> w280
              tunnel: w282 -> [w290 w293]
              frame False {
              }
              frame True {
                n116 = call "Shuffle 1D Array.vim"("array"=i32[] [0, 1, 2, 3, 4, 5, 6, 7, 8, 9, 10, 11, 12, 13, 14, 15, 16, 17, 18, 19, 20, 21, 22, 23, 24, 25, 26, 27, 28, 29] ("Array")) -> ("shuffled array"=w291:i32[])  [unwired: 4 in]
                n117 = Bundle By Name(cluster=w293, "Shuffled Array (Matrix Row Idxs)"=w291) -> (w292:T2)
              }
            }
            n118 = Unbundle By Name(w280) -> ("Output Text File Reference"=w250:refnum<file>)
            n119 = Unbundle By Name(w280) -> ("Sound ID Combination Matrix"=w251:u8[][])
            n120 = Unbundle By Name(w280) -> ("Sound Name Combination Matrix"=w252:string[][])
            n121 = Unbundle By Name(w280) -> ("Sound Data Combination Matrix"=w258:waveform(dbl)[][])
            n122 = Unbundle By Name(w280) -> ("Shuffled Array (Matrix Row Idxs)"=w260:i32[])
            n123 = Unbundle By Name(w280) -> ("Repetitions idx"=w264:i32)
            n124 = Unbundle By Name(w280) -> ("#Sound Total Combinations"=w263:i32)
            n125 = Unbundle By Name(w280) -> ("Combination idx"=w259:i32)
            n126 = Multiply(x=w264, y=w263) -> (x*y=w262:i32)
            n127 = Increment(x=w259) -> (x+1=w267:i32)
            n128 = Add(x=w262, y=w267) -> (x+y=w261:i32)
            "Trial" <- w261
            n129 = global write "global.vi" "Trial"(w261) -> ()
            n130 = Index Array(array=w260, index=w259) -> (element=w253:i32)
            n131 = Index Array(array=w252, index (row)=w253, index (col)=0) -> (element=→"Sound 1":string)
            n132 = Index Array(array=w252, index (row)=w253, index (col)=1) -> (element=→"Sound 2":string)
            n133 = Index Array(array=w258, index (row)=1, index (col)=w253) -> (element=w245:waveform(dbl))
            n134 = Index Array(array=w258, index (row)=0, index (col)=w253) -> (element=w246:waveform(dbl))
            n135 = Index Array(array=w251, index (row)=w253, index (col)=0 ("disabled index (col)")) -> (element=w254:u8)
            n136 = Index Array(array=w251, index (row)=w253, index (col)=1) -> (element=w255:u8)
            n137 = Number To Decimal String(number=w254) -> (decimal integer string=w274:string)  [unwired: 1 in]
            n138 = Number To Decimal String(number=w255) -> (decimal integer string=w275:string)  [unwired: 1 in]
            n139 = Concatenate Strings(w274, "\t" ("string"), w275, "\t" ("string")) -> (w276:string)
            n140 = Write to Text File(file (use dialog)=w250, text=w276) -> (refnum out=w249:refnum<file>)  [unwired: 2 in, 2 out]
            n141 = Bundle By Name(cluster=w280, "Output Text File Reference"=w249) -> (w248:T2)
            n142 = Bundle By Name(cluster=w248, "Sound 1 Data"=w246) -> (w247:T2)
            n143 = Bundle By Name(cluster=w247, "Sound 2 Data"=w245) -> (w279:T2)
          }
          frame True {
          }
        }
      }
      frame "Wait S1" {
        w302 = "Wait..." ("Sound number")
        # "Wait S1 - Waiting state before the first sound playing."
        n144 = local write "Section 1"(FALSE ("Section 1")) -> ()
        n145 = local write "Section 3"(TRUE ("Section 3")) -> ()
        n146 = local write "Section 4"(FALSE ("Section 4")) -> ()
        n147 = local write "Section 5"(FALSE ("Section 5")) -> ()
        n148 = local read "Waiting time 1 [ms]"() -> (w297:i32)
        n149 = global write "global.vi" "Red Light"(TRUE ("Red Light")) -> ()
        n150 = global write "global.vi" "Green Light"(FALSE ("Red Light")) -> ()
        n151 = node-c288() -> (w312:T6)  [unwired: 4 in]
        n152 = To Double Precision Float(number=w297) -> (double precision float=w298:dbl)
        n153 = timed-loop {
          timing: w312 -> [_]
          timing-out: [_] -> w311
          i -> [w321]
          stop <- w319 stop-if-true
          n154 = node-c288() -> (w324:i64)  [unwired: 1 in]
          n155 = To Long Integer(number=w324) -> (32bit integer=w322:i32)
          n156 = Multiply(x=w322, y=w321) -> (x*y=w323:i32)
          n157 = Subtract(x="Waiting time 1 [ms]", y=w323) -> (x-y=→"Remaining Time [ms]" →"Remaining time":i32)
          n158 = Greater Or Equal?(x=w323, y="Waiting time 1 [ms]") -> (x >= y?=w320:bool)
          n159 = local read "stop"() -> (w318:bool)
          n160 = node-c288() -> ()  [unwired: 1 in, 1 out]
          n161 = Or(x=w320, y=w318) -> (x .or. y?=w319:bool)
        }
        n162 = property on="Remaining time" class="Slide (strict)"("Scale.Maximum"=w298) -> ()  [unwired: 2 in, 2 out]
        n163 = global write "global.vi" "Repeat Trial"(FALSE ("Repeat Trial")) -> ()
        n164 = property on="Remaining time" class="Slide (strict)"("Fill Color"=u32 3381759) -> ()  [unwired: 2 in, 2 out]
        n165 = local write "Sound number"(w302) -> ()
        n166 = global write "global.vi" "Sound number"(w302) -> ()
        n167 = node-c288(w311) -> ()  [unwired: 1 out]
        n168 = local read "Waiting time 1 [ms]"() -> (w299:i32)
        n169 = event shown="[1] Timeout" {
          selector: _ -> [_ _]
          dyn-events: _ -> [_ _]
          timeout: w299 -> [_ _]
          tunnel: [State."Cleanup" ("States") State."Play Sound 1" ("States")] -> w305
          event "stop": Value Change {
            n170 = event-data() -> ()  [unwired: 1 in, 1 out]
          }
          event Timeout {
            n171 = event-data() -> ()  [unwired: 1 in, 1 out]
          }
        }
      }
      frame "Play Sound 1" {
        w340 = "Sound 1." ("Sound number")
        # "Play sound 1 - Play first sound."
        n172 = local read "Sound Duration [s]"() -> (w341:dbl)
        n173 = node-c288() -> (w344:T6)  [unwired: 4 in]
        n174 = timed-loop {
          timing: w344 -> [_]
          timing-out: [_] -> w343
          i -> [w349]
          stop <- w354 stop-if-true
          n175 = node-c288() -> (w352:i64)  [unwired: 1 in]
          n176 = local read "Sound Duration [s]"() -> (w359:dbl)
          n177 = To Long Integer(number=w352) -> (32bit integer=w350:i32)
          n178 = Multiply(x=w350, y=w349) -> (x*y=w351:i32)
          n179 = To Long Integer(number=w359) -> (32bit integer=w348:i32)
          n180 = Multiply(x=w348, y=1000) -> (x*y=w353:i32)
          n181 = Subtract(x=w353, y=w351) -> (x-y=w357:i32)
          n182 = local write "Remaining Time [ms]"(w357) -> ()
          n183 = local write "Remaining time"(w357) -> ()
          n184 = local read "stop"() -> (w356:bool)
          n185 = Greater Or Equal?(x=w351, y=w353) -> (x >= y?=w355:bool)
          n186 = node-c288() -> ()  [unwired: 1 in, 1 out]
          n187 = Or(x=w356, y=w355) -> (x .or. y?=w354:bool)
        }
        n188 = Multiply(x=w341, y=1000.0) -> (x*y=w342:dbl)
        n189 = property on="Remaining time" class="Slide (strict)"("Scale.Maximum"=w342) -> ()  [unwired: 2 in, 2 out]
        n190 = Unbundle By Name(w335) -> ("Audio Task ID"=w336:T3)
        n191 = Unbundle By Name(w335) -> ("Sound 1 Data"=w337:waveform(dbl))
        n192 = call-poly <vilib>:"Sound Output Write.vi"("data"=w337, "task ID"=w336) -> ("task ID out"=w333:T3)  [unwired: 8 in, 1 out]
        n193 = Bundle By Name(cluster=w335, "Audio Task ID"=w333) -> (w334:T2)
        n194 = property on="Remaining time" class="Slide (strict)"("Fill Color"=u32 16759921) -> ()  [unwired: 2 in, 2 out]
        n195 = node-c288(w343) -> ()  [unwired: 1 out]
        n196 = local write "Sound number"(w340) -> ()
        n197 = global write "global.vi" "Sound number"(w340) -> ()
        n198 = local read "Sound Duration [s]"() -> (w332:dbl)
        n199 = To Long Integer(number=w332) -> (32bit integer=w331:i32)
        n200 = event shown="[1] Timeout" {
          selector: _ -> [_ _]
          dyn-events: _ -> [_ _]
          timeout: w331 -> [_ _]
          tunnel: [State."Cleanup" ("States") State."Wait S2" ("States")] -> w345
          event "stop": Value Change {
            n201 = event-data() -> ()  [unwired: 1 in, 1 out]
          }
          event Timeout {
            n202 = event-data() -> ()  [unwired: 1 in, 1 out]
          }
        }
      }
      frame "Wait S2" {
        w372 = "Wait..." ("Sound number")
        # "Wait S2 - Waiting state before the second sound playing."
        n203 = local read "Waiting time 2 [ms]"() -> (w367:i32)
        n204 = node-c288() -> (w374:T6)  [unwired: 4 in]
        n205 = To Double Precision Float(number=w367) -> (double precision float=w368:dbl)
        n206 = property on="Remaining time" class="Slide (strict)"("Scale.Maximum"=w368) -> ()  [unwired: 2 in, 2 out]
        n207 = timed-loop {
          timing: w374 -> [_]
          timing-out: [_] -> w373
          i -> [w381]
          stop <- w387 stop-if-true
          n208 = node-c288() -> (w385:i64)  [unwired: 1 in]
          n209 = To Long Integer(number=w385) -> (32bit integer=w382:i32)
          n210 = Multiply(x=w382, y=w381) -> (x*y=w386:i32)
          n211 = Subtract(x="Waiting time 2 [ms]", y=w386) -> (x-y=w383:i32)
          n212 = local write "Remaining Time [ms]"(w383) -> ()
          n213 = local write "Remaining time"(w383) -> ()
          n214 = Greater Or Equal?(x=w386, y="Waiting time 2 [ms]") -> (x >= y?=w384:bool)
          n215 = local read "stop"() -> (w388:bool)
          n216 = node-c288() -> ()  [unwired: 1 in, 1 out]
          n217 = Or(x=w384, y=w388) -> (x .or. y?=w387:bool)
        }
        n218 = property on="Remaining time" class="Slide (strict)"("Fill Color"=u32 3381759) -> ()  [unwired: 2 in, 2 out]
        n219 = local write "Sound number"(w372) -> ()
        n220 = global write "global.vi" "Sound number"(w372) -> ()
        n221 = node-c288(w373) -> ()  [unwired: 1 out]
        n222 = local read "Waiting time 2 [ms]"() -> (w369:i32)
        n223 = event shown="[1] Timeout" {
          selector: _ -> [_ _]
          dyn-events: _ -> [_ _]
          timeout: w369 -> [_ _]
          tunnel: [State."Cleanup" ("States") State."Play Sound 2" ("States")] -> w370
          event "stop": Value Change {
            n224 = event-data() -> ()  [unwired: 1 in, 1 out]
          }
          event Timeout {
            n225 = event-data() -> ()  [unwired: 1 in, 1 out]
          }
        }
      }
      frame "Play Sound 2" {
        w404 = "Sound 2." ("Sound number")
        # "Play sound 2 - Play second sound."
        n226 = local read "Sound Duration [s]"() -> (w405:dbl)
        n227 = node-c288() -> (w409:T6)  [unwired: 4 in]
        n228 = Multiply(x=w405, y=1000.0) -> (x*y=w406:dbl)
        n229 = property on="Remaining time" class="Slide (strict)"("Scale.Maximum"=w406) -> ()  [unwired: 2 in, 2 out]
        n230 = timed-loop {
          timing: w409 -> [_]
          timing-out: [_] -> w408
          i -> [w419]
          stop <- w421 stop-if-true
          n231 = node-c288() -> (w417:i64)  [unwired: 1 in]
          n232 = To Long Integer(number=w417) -> (32bit integer=w418:i32)
          n233 = local read "Sound Duration [s]"() -> (w425:dbl)
          n234 = Multiply(x=w418, y=w419) -> (x*y=w415:i32)
          n235 = To Long Integer(number=w425) -> (32bit integer=w414:i32)
          n236 = Multiply(x=w414, y=1000) -> (x*y=w416:i32)
          n237 = Subtract(x=w416, y=w415) -> (x-y=w423:i32)
          n238 = local write "Remaining Time [ms]"(w423) -> ()
          n239 = local write "Remaining time"(w423) -> ()
          n240 = local read "stop"() -> (w420:bool)
          n241 = Greater Or Equal?(x=w415, y=w416) -> (x >= y?=w422:bool)
          n242 = node-c288() -> ()  [unwired: 1 in, 1 out]
          n243 = Or(x=w420, y=w422) -> (x .or. y?=w421:bool)
        }
        n244 = Unbundle By Name(w398) -> ("Audio Task ID"=w400:T3)
        n245 = Unbundle By Name(w398) -> ("Sound 2 Data"=w401:waveform(dbl))
        n246 = call-poly <vilib>:"Sound Output Write.vi"("data"=w401, "task ID"=w400) -> ("task ID out"=w399:T3)  [unwired: 8 in, 1 out]
        n247 = property on="Remaining time" class="Slide (strict)"("Fill Color"=u32 16759921) -> ()  [unwired: 2 in, 2 out]
        n248 = Bundle By Name(cluster=w398, "Audio Task ID"=w399) -> (w397:T2)
        n249 = local write "Sound number"(w404) -> ()
        n250 = global write "global.vi" "Sound number"(w404) -> ()
        n251 = node-c288(w408) -> ()  [unwired: 1 out]
        n252 = local read "Sound Duration [s]"() -> (w394:dbl)
        n253 = local write "User Choice"("" ("User Choice")) -> ()
        n254 = To Long Integer(number=w394) -> (32bit integer=w395:i32)
        n255 = event shown="[1] Timeout" {
          selector: _ -> [_ _]
          dyn-events: _ -> [_ _]
          timeout: w395 -> [_ _]
          tunnel: [State."Cleanup" ("States") State."Wait for Answer" ("States")] -> w396
          event "stop": Value Change {
            n256 = event-data() -> ()  [unwired: 1 in, 1 out]
          }
          event Timeout {
            n257 = event-data() -> ()  [unwired: 1 in, 1 out]
          }
        }
      }
      frame "Wait for Answer" {
        w450 = "Answer, please:" ("Sound number")
        # "Wait for Answer - Wait for the answer of the user."
        n258 = Unbundle By Name(w436) -> ("Output Text File Reference"=w445:refnum<file>)
        n259 = Unbundle By Name(w436) -> ("Combination idx"=w433:i32)
        n260 = Unbundle By Name(w436) -> ("#Sound Total Combinations"=w442:i32)
        n261 = Unbundle By Name(w436) -> ("Repetitions idx"=w432:i32)
        n262 = Increment(x=w433) -> (x+1=w440:i32)
        n263 = Equal?(x=w440, y=w442) -> (x = y?=w441:bool)
        n264 = case shown="True" w441 {
          tunnel: w432 -> [w455 w457]
          tunnel: [w455 w456] -> w435
          frame False {
          }
          frame True {
            n265 = Increment(x=w457) -> (x+1=w456:i32)
          }
        }
        n266 = while {
          tunnel: [w472] -> w444
          tunnel: w445 -> [w471]
          tunnel: [w464] -> w443
          tunnel: w435 -> [w463]
          tunnel: [w462] -> w434
          tunnel: w433 -> [w461]
          tunnel: w432 -> [w460]
          tunnel: [w459] -> w431
          stop <- w465 stop-if-true
          n267 = global read "global.vi" "Choice 1"() -> (w470:bool)
          n268 = global read "global.vi" "Choice 2"() -> (w469:bool)
          n269 = global read "global.vi" "Choice Equal"() -> (w468:bool)
          n270 = global read "global.vi" "Repeat Trial"() -> (w458:bool)
          n271 = case shown="False" w470 {
            tunnel: [w482 w493] -> w472
            tunnel: w469 -> [_ w492]
            tunnel: w471 -> [w481 w491]
            tunnel: w468 -> [_ w490]
            tunnel: [State."Start New Trial" ("States") w489] -> w464
            tunnel: w463 -> [w477 w488]
            tunnel: [w477 w487] -> w462
            tunnel: w461 -> [w476 w486]
            tunnel: w460 -> [_ w485]
            tunnel: [w475 w484] -> w459
            tunnel: w458 -> [_ w483]
            frame True {
              n272 = Write to Text File(file (use dialog)=w481, text="1\n") -> (refnum out=w482:refnum<file>)  [unwired: 2 in, 2 out]
              n273 = local write "User Choice"("Sound 1" ("User Choice")) -> ()
              n274 = Increment(x=w476) -> (x+1=w475:i32)
            }
            frame False {
              n275 = case shown="False" w492 {
                tunnel: [w503 w533] -> w493
                tunnel: w491 -> [w502 w532]
                tunnel: w490 -> [w501 _]
                tunnel: [w500 State."Start New Trial" ("States")] -> w489
                tunnel: w488 -> [w499 w528]
                tunnel: [w498 w528] -> w487
                tunnel: w486 -> [w497 w527]
                tunnel: w485 -> [w496 _]
                tunnel: [w495 w526] -> w484
                tunnel: w483 -> [w494 _]
                frame False {
                  n276 = case shown="False" w501 {
                    tunnel: [w511 w524] -> w503
                    tunnel: w502 -> [w511 w523]
                    tunnel: [w504 State."Start New Trial" ("States")] -> w500
                    tunnel: w499 -> [w508 w520]
                    tunnel: [w505 w520] -> w498
                    tunnel: w497 -> [w509 w519]
                    tunnel: w496 -> [w507 _]
                    tunnel: [w506 w518] -> w495
                    tunnel: w494 -> [w510 _]
                    frame False {
                      n277 = case shown="True" w510 {
                        tunnel: w509 -> [w512 w517]
                        tunnel: w508 -> [_ _]
                        tunnel: w507 -> [w513 w516]
                        tunnel: [w512 w517] -> w506
                        tunnel: [w513 w516] -> w505
                        tunnel: [State."Cleanup" ("States") State."Wait S1" ("States")] -> w504
                        frame False {
                        }
                        frame True {
                        }
                      }
                    }
                    frame True {
                      n278 = Write to Text File(file (use dialog)=w523, text="0\n") -> (refnum out=w524:refnum<file>)  [unwired: 2 in, 2 out]
                      n279 = local write "User Choice"("Equal" ("User Choice")) -> ()
                      n280 = Increment(x=w519) -> (x+1=w518:i32)
                    }
                  }
                }
                frame True {
                  n281 = Write to Text File(file (use dialog)=w532, text="2\n") -> (refnum out=w533:refnum<file>)  [unwired: 2 in, 2 out]
                  n282 = local write "User Choice"("Sound 2" ("User Choice")) -> ()
                  n283 = Increment(x=w527) -> (x+1=w526:i32)
                }
              }
            }
          }
          n284 = Or(x=w470, y=w469) -> (x .or. y?=w474:bool)
          n285 = local read "stop"() -> (w466:bool)
          n286 = Or(x=w474, y=w468) -> (x .or. y?=w473:bool)
          n287 = Or(x=w473, y=w458) -> (x .or. y?=w467:bool)
          n288 = Or(x=w467, y=w466) -> (x .or. y?=w465:bool)
        }
        n289 = Bundle By Name(cluster=w436, "Output Text File Reference"=w444) -> (w439:T2)
        n290 = Bundle By Name(cluster=w439, "Combination idx"=w431) -> (w438:T2)
        n291 = Bundle By Name(cluster=w438, "Repetitions idx"=w434) -> (w437:T2)
        n292 = global write "global.vi" "Red Light"(FALSE ("Red Light")) -> ()
        n293 = global write "global.vi" "Green Light"(TRUE ("Red Light")) -> ()
        n294 = local write "Section 1"(FALSE ("Section 1")) -> ()
        n295 = local write "Section 3"(FALSE ("Section 3")) -> ()
        n296 = local write "Section 4"(TRUE ("Section 4")) -> ()
        n297 = local write "Section 5"(FALSE ("Section 5")) -> ()
        n298 = local write "Sound number"(w450) -> ()
        n299 = global write "global.vi" "Sound number"(w450) -> ()
      }
      frame "Cleanup" {
        w542 = "Protocol finished. " ("Sound number")
        # "Cleanup - Clean the variable and indicator values before closing."
        n300 = local write "stop"(FALSE ("stop")) -> ()
        n301 = global write "global.vi" "stop"(TRUE ("stop")) -> ()
        n302 = global write "global.vi" "Start"(FALSE ("Start")) -> ()
        n303 = global write "global.vi" "Red Light"(FALSE ("Red Light")) -> ()
        n304 = global write "global.vi" "Green Light"(FALSE ("Red Light")) -> ()
        n305 = Unbundle By Name(w536) -> ("Output Text File Reference"=w534:refnum<file>)
        n306 = Unbundle By Name(w536) -> ("Audio Task ID"=w535:T3)
        n307 = Close File(refnum=w534) -> ()  [unwired: 1 in, 2 out]
        n308 = call <vilib>:"Sound Output Clear.vi"("task ID"=w535) -> ()  [unwired: 10 in, 1 out]
        n309 = local write "Sound number"(w542) -> ()
        n310 = global write "global.vi" "Sound number"(w542) -> ()
        n311 = local write "Section 1"(FALSE ("Section 1")) -> ()
        n312 = local write "Section 3"(FALSE ("Section 3")) -> ()
        n313 = local write "Section 4"(FALSE ("Section 4")) -> ()
        n314 = local write "Section 5"(TRUE ("Section 5")) -> ()
      }
      frame "Exit" {
        w553 = TRUE  # Stop Loop?
        w554 = State."Exit"  # (Value Not Used)
        # "Exit - Exit the application."
        n315 = Unbundle By Name(w551) -> ("User VI Reference"=w550:refnum<vi>)
        n316 = Close Reference(reference=w550) -> ()  [unwired: 1 in, 1 out]
      }
    }
    n317 = Or(x=w6, y=w8) -> (x .or. y?=w7:bool)
  }
  n318 = call <vilib>:"Simple Error Handler.vi"("error in (no error)"=w4) -> ("error out"=w3:errorcluster)  [unwired: 4 in, 4 out]
  n319 = disable-structure shown="RUN_TIME_ENGINE==True" {
    disable-tunnel: w3 -> [_ _]
    frame condition #0 (active) {
    }
    frame condition #1 {
      # "Call Quit LabVIEW if running as a built application."
      n320 = Quit LabVIEW() -> ()  [unwired: 1 in]
    }
  }
